vi "Create_Object.vi"(8 "error in (no error)":errorcluster, 9 "Terminal Map in":map{string, T1}(c390), 10 "vi refnum in":refnum<vi>, 11 "String Constant in":refnum<class "String Constant.lvclass">) -> (0 "error out":errorcluster, 1 "Terminal Map Out":map{string, T1}(c390), 3 "String Constant out":refnum<class "String Constant.lvclass">)   [LabVIEW 2025, in "String Constant.lvclass"]
uses:
  String Constant.lvclass
  home/jake/Documents/github/LVGPT/LabVIEW/VIs/Classes/Node/Node.lvclass
  Terminal.ctl
  Node/Node.lvclass/Node.ctl
  Constant.lvclass
  Node/Node.lvclass
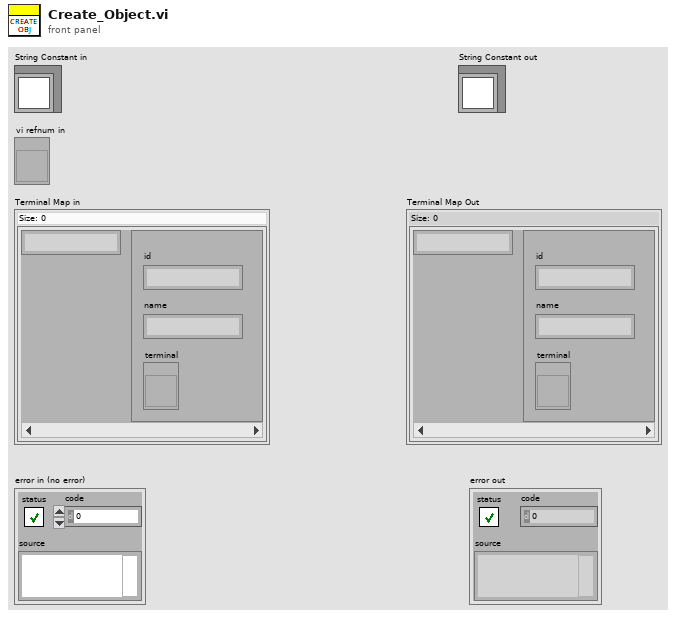
[diagram p1: front panel]
types:
  T1 = typedef "Terminal.ctl" = cluster{"id":string, "name":string, "terminal":refnum<vi>}
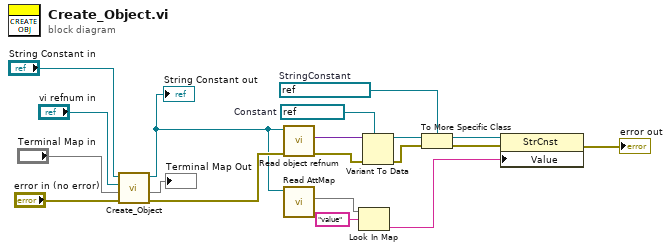
[diagram p0: block diagram]
diagram:
  w10 = refnum<vi> refnum  # StringConstant
  w12 = refnum<vi> refnum  # Constant
  n1 = call-parent "Create_Object.vi"("error in (no error)"="error in (no error)", "Terminal Map in"="Terminal Map in", "vi refnum in"="vi refnum in", "Constant in"="String Constant in") -> ("error out"=w15:errorcluster, "Terminal Map Out"=→"Terminal Map Out":map{string, T1}, "Constant out"=w2:refnum<class "String Constant.lvclass">)  [unwired: 5 in]
  "String Constant out" <- w2
  n2 = call-dynamic "Read object refnum.vi"("error in (no error)"=w15, "Node in"=w2) -> ("error out"=w9:errorcluster, "object refnum"=w13:variant)  [unwired: 7 in, 1 out]
  n3 = call "Read AttMap.vi"("Node in"=w2) -> ("AttMap"=w5:map{string, string})  [unwired: 8 in, 2 out]
  n4 = Look In Map(map=w5, key="value") -> (value=w3:string)  [unwired: 1 in, 1 out]
  n5 = Variant To Data(error in=w9, type=w12, Variant=w13) -> (data=w11:refnum<vi>, error out=w8:errorcluster)
  n6 = To More Specific Class(target class=w10, reference=w11, error in=w8) -> (specific class reference=w7:refnum<vi>, error out=w6:errorcluster)
  n7 = property class="StrCnst"(reference=w7, error in=w6, "Value"=w3) -> (error out=→"error out":errorcluster)  [unwired: 1 out]
